vi "run.vi"(11 "sequence task in":refnum<class "sequence task.lvclass">) -> (2 "result":refnum<class "result.lvclass">, 3 "sequence task out":refnum<class "sequence task.lvclass">)   [LabVIEW 2013, in "sequence task.lvclass"]
uses:
  sequence task.lvclass
  result/result.lvclass
  sequence task.lvclass/sequence task.ctl
  task/task.lvclass
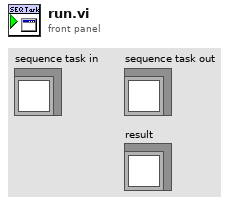
[diagram p1: front panel]
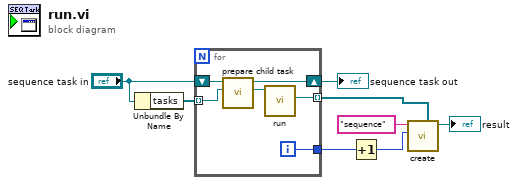
[diagram p0: block diagram]
diagram:
  n1 = Unbundle By Name("sequence task in") -> ("tasks"=w8:refnum<class "task.lvclass">[])
  n2 = for {
    tunnel: w8 -> [w9] mode=indexing
    tunnel: [w14] -> w6 mode=indexing
    tunnel: [w13] -> w5
    shift-right: [w11] -> w2
    shift-left: "sequence task in" -> [w12]
    i -> [w13]
    n3 = call "prepare child task.vi"("child task in"=w9, "task in"=w12) -> ("child task out"=w10:refnum<class "task.lvclass">, "task out"=w11:refnum<class "sequence task.lvclass">)  [unwired: 8 in]
    n4 = call-dynamic "run.vi"("task in"=w10) -> ("result"=w14:refnum<class "result.lvclass">)  [unwired: 9 in, 1 out]
  }
  "sequence task out" <- w2
  n5 = Increment(x=w5) -> (x+1=w4:i32)
  n6 = call "create.vi"("subresults"=w6, "data"=w4, "data ID"="sequence") -> ("result out"=→"result":refnum<class "result.lvclass">)  [unwired: 8 in]
